vi "2 update_currents_drift.vi"   [LabVIEW 2011]
doc: "Finds the error of the boats heading versus movement, and attributes that to current. This uses the error between heading and bearing, as well as the Think Frequency, to determine the velocity of the currents. Only the current velocity normal to the boat's heading is found, but this is all that we need to know to shift the goal."
uses:
  2 Typedefs/heading.ctl
  2 Globals/2 Global.vi
types:
  T1 = typedef "heading.ctl" = dbl
  T2 = typedef "Velocity.ctl" = cluster{"East":dbl, "North":dbl}
  T3 = typedef "UTM Location.ctl" = cluster{"UTM Zone":dbl, "Hemisphere":enum16{"North", "South"}, "East":dbl, "North":dbl}
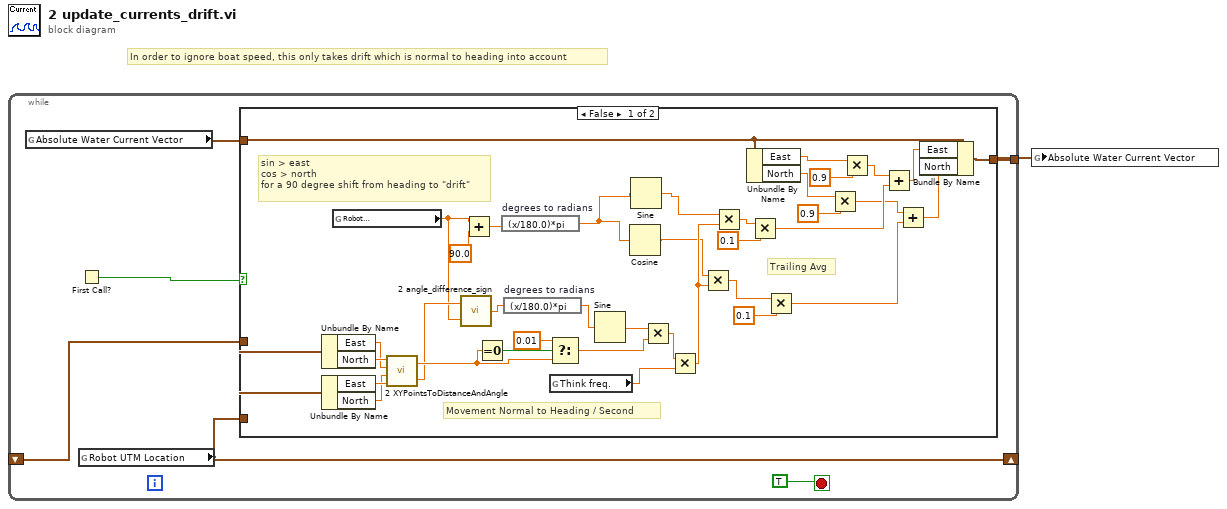
[diagram p0: block diagram]
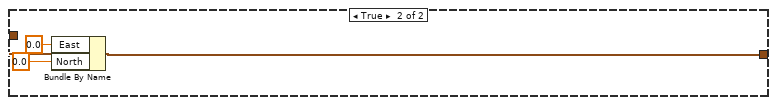
[diagram p2: hidden frame]
diagram:
  # "In order to ignore boat speed, this only takes drift which is normal to heading into account"
  n1 = while {
    tunnel: [w6] -> w1
    shift-right: [w3] -> _
    shift-left: _ -> [w4]
    stop <- TRUE stop-if-true
    n2 = global read "2 Global.vi" "Absolute Water Current Vector"() -> (w7:T2)
    n3 = First Call?() -> (First Call?: T/F=w2:bool)
    n4 = global read "2 Global.vi" "Robot UTM Location"() -> (w3:T3)
    n5 = case shown="False" w2 {
      tunnel: w7 -> [w39 w50]
      tunnel: [w40 w49] -> w6
      tunnel: w4 -> [w46 _]
      tunnel: w3 -> [w45 _]
      frame False {
        # "Trailing Avg"
        # "sin > east\ncos > north\nfor a 90 degree shift from heading to \"drift\""
        # "Movement Normal to Heading / Second"
        n6 = Unbundle By Name(w45) -> ("East"=w16:dbl, "North"=w19:dbl)
        n7 = Unbundle By Name(w46) -> ("East"=w21:dbl, "North"=w20:dbl)
        n8 = global read "2 Global.vi" "Robot\nHeading"() -> (w9:T1)
        n9 = call "2 XYPointsToDistanceAndAngle.vi"("East 2"=w21, "North 2"=w20, "East 1"=w16, "North 1"=w19) -> ("Angle Diff"=w17:dbl, "Distance"=w18:dbl)
        n10 = call "2 angle_difference_sign.vi"("Angle 2"=w9, "Angle 1"=w17) -> ("Difference"=w14:dbl)
        n11 = Add(x=w9, y=T1 90.0) -> (x+y=w10:T1)
        n12 = Equal To 0?(x=w18) -> (x = 0?=w24:bool)
        n13 = expression code="(x/180.0)*pi" "degrees to radians"(w10) -> (w12:T1)
        n14 = expression code="(x/180.0)*pi" "degrees to radians"(w14) -> (w15:dbl)
        n15 = Select(t=0.01, s=w24, f=w18) -> (s? t:f=w22:dbl)
        n16 = global read "2 Global.vi" "Think freq."() -> (w42:dbl)
        n17 = Sine(x=w15) -> (sin(x)=w44:dbl)
        n18 = Cosine(x=w12) -> (cos(x)=w13:T1)
        n19 = Sine(x=w12) -> (sin(x)=w11:T1)
        n20 = Multiply(x=w44, y=w22) -> (x*y=w43:dbl)
        n21 = Multiply(x=w43, y=w42) -> (x*y=w41:dbl)
        n22 = Multiply(x=w13, y=w41) -> (x*y=w35:T1)
        n23 = Multiply(x=w11, y=w41) -> (x*y=w38:T1)
        n24 = Unbundle By Name(w39) -> ("East"=w33:dbl, "North"=w31:dbl)
        n25 = Multiply(x=w38, y=T1 0.1) -> (x*y=w29:T1)
        n26 = Multiply(x=w35, y=T1 0.1) -> (x*y=w27:T1)
        n27 = Multiply(x=w31, y=T1 0.9) -> (x*y=w28:T1)
        n28 = Multiply(x=w33, y=T1 0.9) -> (x*y=w30:T1)
        n29 = Add(x=w30, y=w29) -> (x+y=w26:T1)
        n30 = Add(x=w28, y=w27) -> (x+y=w25:T1)
        n31 = Bundle By Name(cluster=w39, "East"=w26, "North"=w25) -> (w40:T2)
      }
      frame True {
        n32 = Bundle By Name(cluster=w50, "East"=0.0, "North"=0.0) -> (w49:T2)
      }
    }
  }
  n33 = global write "2 Global.vi" "Absolute Water Current Vector"(w1) -> ()
